vi "convertToKeyValuePair_1DArray.vi"(8 "error in (no error)":errorcluster, 9 "presicion (0)":u8, 10 "value":dbl[](array[numeric]), 11 "name":string) -> (0 "error out":errorcluster, 3 "string converted":string)   [LabVIEW 2018]
doc: "Convert a 1-dimension array into a key value pair as string."
uses:
  convertToKeyValuePair_string.vi
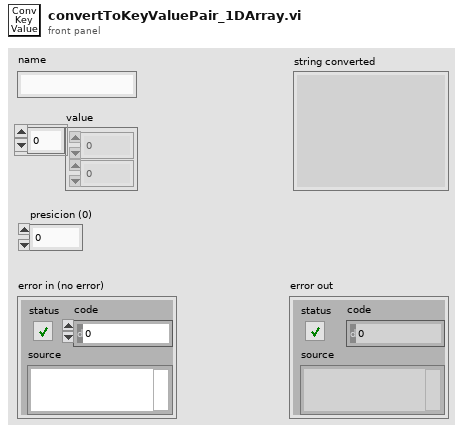
[diagram p1: front panel]
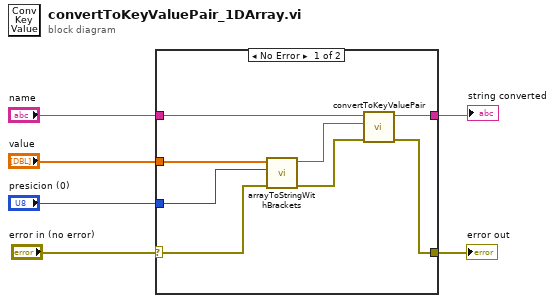
[diagram p0: block diagram]
diagram:
  n1 = case shown="No Error" "error in (no error)" {
    selector: "error in (no error)" -> [w8 w15]
    tunnel: "value" -> [w11 _]
    tunnel: "name" -> [w13 _]
    tunnel: "presicion (0)" -> [w10 _]
    tunnel: [w12 w15] -> w2
    tunnel: [w14 _] -> w1
    frame No Error {
      n2 = call "arrayToStringWithBrackets.vi"("error in (no error)"=w8, "presicion (0)"=w10, "value"=w11) -> ("error out"=w7:errorcluster, "String"=w9:string)  [unwired: 7 in]
      n3 = call-poly "convertToKeyValuePair.vi"("error in (no error)"=w7, "value"=w9, "name"=w13) -> ("error out"=w12:errorcluster, "string converted"=w14:string)  [unwired: 7 in]
    }
    frame Error {
    }
  }
  "error out" <- w2
  "string converted" <- w1
